vi "Curve fit V1.vi"(11 "x":dbl) -> (3 "res":dbl)   [LabVIEW 2013]
panel:
  in  "Stop Button":bool
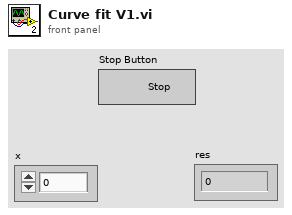
[diagram p1: front panel]
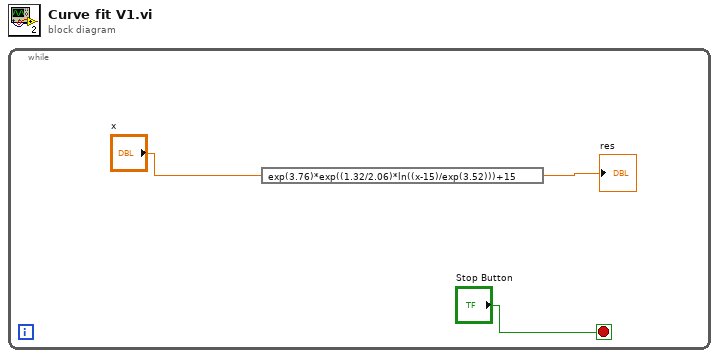
[diagram p0: block diagram]
diagram:
  n1 = while {
    stop <- "Stop Button" stop-if-true
    n2 = expression code="exp(3.76)*exp((1.32/2.06)*ln((x-15)/exp(3.52)))+15"("x") -> (→"res":dbl)
  }
